vi "Method_Const.vi"(4 "Value":i16, 5 "A":T1) -> (1 "Result":T1)   [LabVIEW 2021, in "EXOR_I16.lvclass"]
uses:
  EXOR_I16.lvclass
  Abs_Type.ctl
  Abs_Types/I16 Integer/Abs_I16 Integer.lvclass
  C:/Program Files (x86)/National Instruments/LabVIEW 2021/vi.lib/TSA/Abstract Data Classes/Abs_Types/Numeric/Abs_Numeric.lvclass
  C:/TSA/LV_Abstract/Source/Functions/Support/Function/Two Terminal/I16/AbsFunc_Two Term_I16.lvclass
  C:/Program Files (x86)/National Instruments/LabVIEW 2021/vi.lib/TSA/Abstract Data Classes/Abs_Types/I16 Integer/Abs_I16 Integer.lvclass
  Support/Function/Two Terminal/I16/AbsFunc_Two Term_I16.lvclass/AbsFunc_Two Term_I16.ctl
  Support/Function/Two Terminal/I16/Properties/Write Numeric A.vi
  Support/Function/Two Terminal/I16/Properties/Write Numeric B.vi
  Constants/Support/I16/Const_I16.lvclass
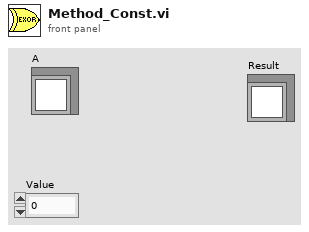
[diagram p1: front panel]
types:
  T1 = typedef "EXOR_I16.lvclass/Abs_Type.ctl" = refnum<class "Abs_I16 Integer.lvclass">
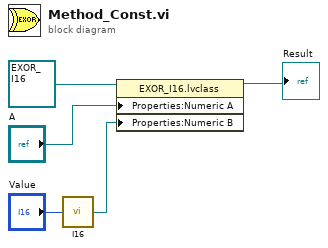
[diagram p0: block diagram]
diagram:
  n1 = call "I16.vi"("Value"="Value") -> ("Constant"=w2:refnum<class "Abs_I16 Integer.lvclass">)  [unwired: 4 in]
  n2 = property class="EXOR_I16.lvclass"(reference=refnum<class "EXOR_I16.lvclass"> refnum ("Functions.lvlib:Logic.lvlib:AND.lvclass"), "Properties:Numeric A"="A", "Properties:Numeric B"=w2) -> (reference out=→"Result":refnum<class "EXOR_I16.lvclass">)  [unwired: 1 in, 1 out]
